vi "VRM.Hold.vi"(6 "Axis":T1=enum."Z", 8 "error in (no error)":errorcluster, 11 "Instrument.VRM in":refnum<class "Instrument.OxfordVRM.lvclass">) -> (0 "error out":errorcluster, 2 "Response":string[](array[string]), 3 "Instrument.VRM out":refnum<class "Instrument.OxfordVRM.lvclass">)   [LabVIEW 2019, in "Instrument.OxfordVRM.lvclass"]
uses:
  Instrument.OxfordVRM.lvclass
  Typedefs/VRM Magnet Axis--Enum.ctl
  <instrlib>/Mercury iXX/Public/Libraries/Magnet/Controls/PSU Actions.ctl
  <instrlib>/Mercury iXX/Public/Libraries/Magnet.lvlib
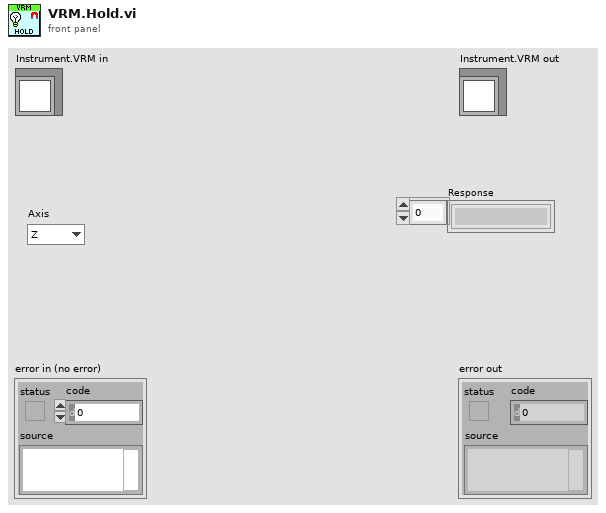
[diagram p1: front panel]
types:
  T1 = typedef "Instrument.OxfordVRM.lvclass/VRM Magnet Axis--Enum.ctl" = enum16{"X", "Y", "Z", "ALL"}
  T2 = typedef "Mercury iXX.lvlib/Magnet.lvlib/PSU Actions.ctl" = string
  T3 = typedef "Instrument.Cryostat.lvclass/Magnet Axis--Enum.ctl" = enum16{"X", "Y", "Z"}
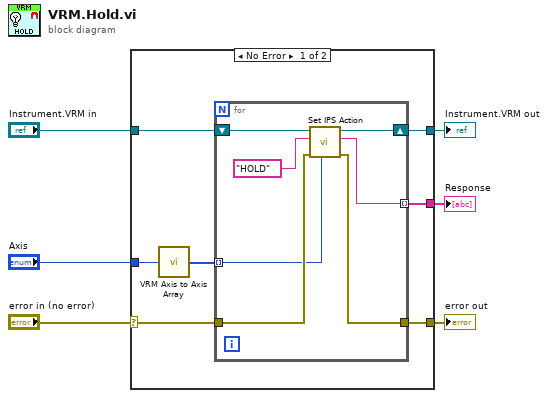
[diagram p0: block diagram]
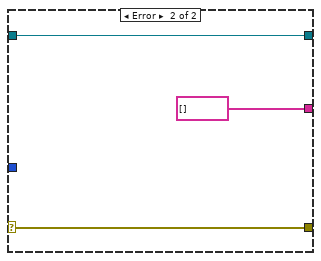
[diagram p2: hidden frame]
diagram:
  n1 = case shown="No Error" "error in (no error)" {
    selector: "error in (no error)" -> [w12 w23]
    tunnel: [w9 w23] -> w5
    tunnel: [w10 w22] -> w3
    tunnel: "Instrument.VRM in" -> [w13 w22]
    tunnel: "Axis" -> [w11 _]
    tunnel: [w8 string[] []] -> w1
    frame No Error {
      n2 = call "VRM Axis to Axis Array.vi"("Axis"=w11) -> ("Axis Array"=w7:T3[])
      n3 = for {
        tunnel: w7 -> [w18] mode=indexing
        shift-right: [w17] -> w10
        shift-left: w13 -> [w20]
        tunnel: [w14] -> w8 mode=indexing
        tunnel: w12 -> [w19]
        tunnel: [w15] -> w9
        n4 = call "Set IPS Action.vi"("Axis"=w18, "error in (no error)"=w19, "PSU Act Stat"=T2 "HOLD", "Instrument.OxfordVRM in"=w20) -> ("error out"=w15:errorcluster, "Response"=w14:string, "Instrument.OxfordVRM out"=w17:refnum<class "Instrument.OxfordVRM.lvclass">)  [unwired: 5 in]
      }
    }
    frame Error {
    }
  }
  "error out" <- w5
  "Instrument.VRM out" <- w3
  "Response" <- w1
